vi "Light_Sensor_LED_BB.vi"   [LabVIEW 2012]
types:
  T1 = typedef "BotSpeak_Control.ctl" = cluster{"Address":string, "Reply EOF":string, "Hardware":string, "Retries":i8, "Timeout":i32}
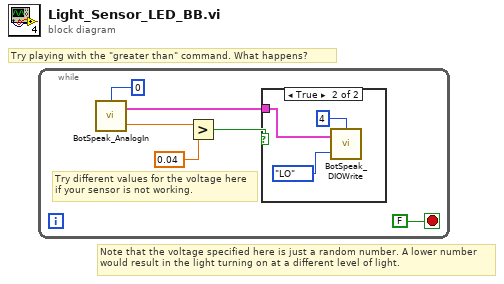
[diagram p0: block diagram]
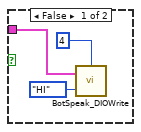
[diagram p2: hidden frame]
diagram:
  # "Try playing with the \"greater than\" command. What happens?"
  # "Note that the voltage specified here is just a random number. A lower number would result in the light turning on at a different level of light."
  n1 = while {
    stop <- FALSE stop-if-true
    # "Try different values for the voltage here if your sensor is not working."
    n2 = call <userlib>:"BotSpeak_AnalogIn.vi"("A/D Channel"=u8 0) -> ("voltage"=w4:dbl, "Bot Settings"=w5:T1)  [unwired: 2 in]
    n3 = Greater?(x=w4, y=0.04) -> (0:w2:bool)
    n4 = case shown="True" w2 {
      tunnel: w5 -> [w7 w10]
      frame False {
        n5 = call <userlib>:"BotSpeak_DIOWrite.vi"("State"=enum32{"LO", "HI"}."HI", "Bot Settings"=w7, "DIO Line"=u32 4) -> ()  [unwired: 2 out]
      }
      frame True {
        n6 = call <userlib>:"BotSpeak_DIOWrite.vi"("State"=enum32{"LO", "HI"}."LO", "Bot Settings"=w10, "DIO Line"=u32 4) -> ()  [unwired: 2 out]
      }
    }
  }
